vi "Encoded UTF-16LE String to Encoded UTF-8 String.vi"(9 "error in":errorcluster, 10 "Encoded UTF-16LE String":T2) -> (1 "error out":errorcluster, 2 "Encoded UTF-8 String":T1)   [LabVIEW 2020, in "G-Unicode.lvlib"]
uses:
  G-Unicode.lvlib
  Types/Encoded UTF-16LE String.ctl
  Types/Encoded UTF-8 String.ctl
  lib/g_unicode_32.dll
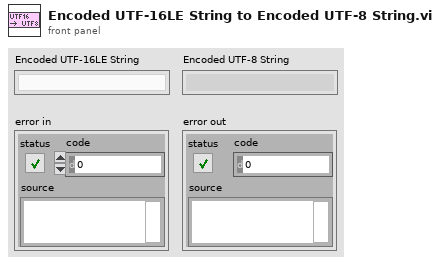
[diagram p1: front panel]
types:
  T1 = typedef "G-Unicode.lvlib/Encoded UTF-8 String.ctl" = string
  T2 = typedef "G-Unicode.lvlib/Encoded UTF-16LE String.ctl" = string
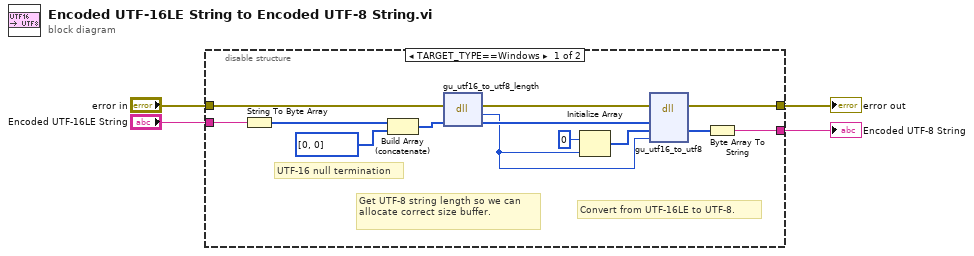
[diagram p0: block diagram]
diagram:
  n1 = disable-structure shown="TARGET_TYPE==Windows" {
    disable-tunnel: "Encoded UTF-16LE String" -> [w8 w18]
    disable-tunnel: [w13 w18] -> w1
    disable-tunnel: "error in" -> [w10 w19]
    disable-tunnel: [w12 w19] -> w2
    frame condition #0 (active) {
      # "UTF-16 null termination"
      # "Convert from UTF-16LE to UTF-8."
      # "Get UTF-8 string length so we can allocate correct size buffer."
      n2 = String To Byte Array(string=w8) -> (unsigned byte array=w6:u8[])
      n3 = Build Array (concatenate)(w6, u8[] [0, 0]) -> (w7:u8[])
      n4 = dll-call lib="C:/github/dataflowg/g-unicode/src/LabVIEW/G-Unicode/lib/g_unicode_*.*" fn="gu_utf16_to_utf8_length"(error in=w10, "utf16"=w7) -> (error out=w11:errorcluster, "length"=w9:i32, "utf16"=w15:u8[])  [unwired: 2 in, 1 out]
      n5 = Initialize Array(u8 0 ("dwFlags"), w9) -> (w16:u8[])
      n6 = dll-call lib="C:/github/dataflowg/g-unicode/src/LabVIEW/G-Unicode/lib/g_unicode_*.*" fn="gu_utf16_to_utf8"(error in=w11, "utf16"=w15, "utf8"=w16, "utf8_length"=w9) -> (error out=w12:errorcluster, "utf8"=w14:u8[])  [unwired: 5 in, 1 out]
      n7 = Byte Array To String(unsigned byte array=w14) -> (string=w13:string)
    }
    frame condition #1 {
    }
  }
  "error out" <- w2
  "Encoded UTF-8 String" <- w1
